vi "Get Cassete codes.vi"(8 "error in (no error)":errorcluster, 11 "Variant":string) -> (0 "error out":errorcluster, 2 "Variant not found":bool, 3 "Cassete code":bool[](array[boolean]))   [LabVIEW 2023]
uses:
  <vilib>/Utility/config.llb/Read Key (I32).vi
  <vilib>/Utility/config.llb/NI_LVConfig.lvlib
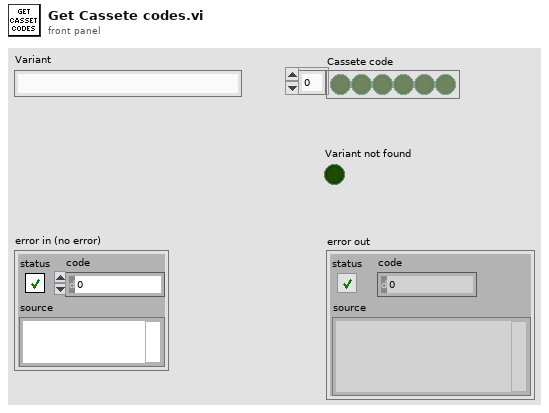
[diagram p1: front panel]
types:
  T1 = typedef "NI_LVConfig.lvlib/Config Data RefNum.ctl" = refnum<k1>
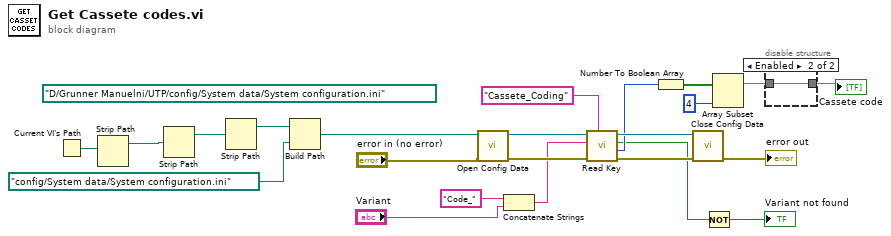
[diagram p0: block diagram]
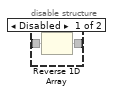
[diagram p2: hidden frame]
diagram:
  (unwired) path "D:/Grunner Manuelni/UTP/config/System data/System configuration.ini" ("configuration file path")
  n1 = Current VI's Path() -> (path=w9:path)
  n2 = Strip Path(path=w9) -> (stripped path=w8:path)  [unwired: 1 out]
  n3 = Strip Path(path=w8) -> (stripped path=w13:path)  [unwired: 1 out]
  n4 = Strip Path(path=w13) -> (stripped path=w12:path)  [unwired: 1 out]
  n5 = Build Path(base path=w12, name or relative path=path "config/System data/System configuration.ini") -> (appended path=w10:path)
  n6 = call <vilib>:"Open Config Data.vi"("error in (no error)"="error in (no error)", "configuration file path"=w10) -> ("error out"=w21:errorcluster, "refnum"=w20:T1)  [unwired: 7 in, 1 out]
  n7 = Concatenate Strings("Code_" ("key"), "Variant") -> (w16:string)
  n8 = call-poly <vilib>:"Read Key.vi"("section"="Cassete_Coding", "error in (no error)"=w21, "key"=w16, "refnum"=w20) -> ("error out"=w18:errorcluster, "value"=w7:i32, "found?"=w2:bool, "refnum out"=w19:T1)  [unwired: 4 in]
  n9 = Number To Boolean Array(number=w7) -> (Boolean array=w5:bool[])
  n10 = call <vilib>:"Close Config Data.vi"("error in (no error)"=w18, "refnum"=w19) -> ("error out"=→"error out":errorcluster)  [unwired: 8 in, 1 out]
  n11 = Not(x=w2) -> (.not. x?=→"Variant not found":bool)
  n12 = Array Subset(array=w5, length=4) -> (w6:bool[])  [unwired: 1 in]
  n13 = disable-structure shown="Enabled" {
    disable-tunnel: w6 -> [w25 w26]
    disable-tunnel: [w24 w26] -> w3
    frame Disabled {
      n14 = Reverse 1D Array(array=w25) -> (reversed array=w24:bool[])
    }
    frame Enabled {
    }
  }
  "Cassete code" <- w3
